vi "Prase XML.vi"() -> ()   [LabVIEW 2020]
uses:
  <vilib>/xml/Close Reference(Node).vi
  <vilib>/xml/Close Reference(NdList).vi
  <vilib>/xml/NI_XML.lvlib
  <resource>/objmgr/DOMUserDefRef.rc
panel:
  out "Test\nConfiguration":T1(array[cluster])
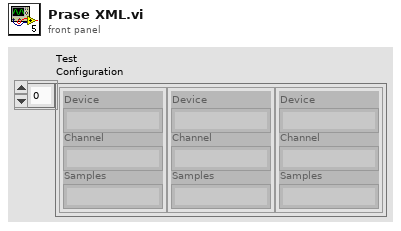
[diagram p1: front panel]
types:
  T1 = cluster{"Device":string, "Channel":string, "Samples":string}[]
  T2 = cluster{"Device":string, "Channel":string, "Samples":string}
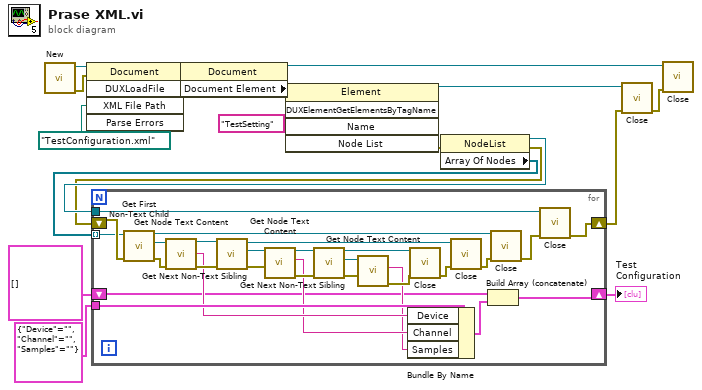
[diagram p0: block diagram]
diagram:
  n1 = call <vilib>:"New.vi"() -> ("error out"=w19:errorcluster, "DOM document out"=w20:refnum<k20>)  [unwired: 1 in, 7 out]
  n2 = invoke class="Document" method="DUXLoadFile"(reference=w20, error in=w19, "XML File Path"=path "TestConfiguration.xml") -> (reference out=w18:refnum<k20>, error out=w17:errorcluster)  [unwired: 2 in, 3 out]
  n3 = property class="Document"(reference=w18, error in=w17) -> (reference out=w6:refnum<k20>, error out=w15:errorcluster, "Document Element"=w7:refnum<k20>)
  n4 = invoke class="Element" method="DUXElementGetElementsByTagName"(reference=w7, error in=w15, "Name"="TestSetting" ("Node Name")) -> (reference out=w8:refnum<k20>, error out=w5:errorcluster, "Node List"=w4:refnum<k20>)  [unwired: 2 in, 2 out]
  n5 = property class="NodeList"(reference=w4, error in=w5) -> (reference out=w11:refnum<k20>, error out=w10:errorcluster, "Array Of Nodes"=w12:refnum<k20>[])
  n6 = for {
    tunnel: w12 -> [w21] mode=indexing
    tunnel: w11 -> [w32]
    shift-right: [w24] -> w1
    shift-left: T1 [] -> [w26]
    shift-right: [w31] -> w3
    shift-left: w10 -> [w23]
    tunnel: T2 {"Device"="", "Channel"="", "Samples"=""} -> [w30]
    n7 = call <vilib>:"Get First Non-Text Child.vi"("error in (no error)"=w23, "node in"=w21) -> ("error out"=w47:errorcluster, "child node"=w48:refnum<k20>, "node out"=w40:refnum<k20>)  [unwired: 7 out]
    n8 = call <vilib>:"Get Node Text Content.vi"("error in (no error)"=w47, "node in"=w48) -> ("error out"=w43:errorcluster, "node text"=w29:string, "node out"=w44:refnum<k20>)  [unwired: 7 out]
    n9 = call <vilib>:"Get Next Non-Text Sibling.vi"("error in (no error)"=w43, "node in"=w44) -> ("error out"=w46:errorcluster, "sibling node"=w45:refnum<k20>, "node out"=w42:refnum<k20>)  [unwired: 7 out]
    n10 = call <vilib>:"Get Node Text Content.vi"("error in (no error)"=w46, "node in"=w45) -> ("error out"=w36:errorcluster, "node text"=w28:string, "node out"=w38:refnum<k20>)  [unwired: 7 out]
    n11 = call <vilib>:"Get Next Non-Text Sibling.vi"("error in (no error)"=w36, "node in"=w38) -> ("error out"=w35:errorcluster, "sibling node"=w34:refnum<k20>, "node out"=w37:refnum<k20>)  [unwired: 7 out]
    n12 = call <vilib>:"Get Node Text Content.vi"("error in (no error)"=w35, "node in"=w34) -> ("error out"=w33:errorcluster, "node text"=w27:string)  [unwired: 8 out]
    n13 = Bundle By Name(cluster=w30, "Device"=w29, "Channel"=w28, "Samples"=w27) -> (w25:T2)
    n14 = call-poly <vilib>:"Close.vi"("error in (no error)"=w33, "node"=w37) -> ("error out"=w41:errorcluster)  [unwired: 7 out]
    n15 = call-poly <vilib>:"Close.vi"("error in (no error)"=w41, "node"=w42) -> ("error out"=w39:errorcluster)  [unwired: 7 out]
    n16 = Build Array (concatenate)(w26, w25) -> (w24:T1)
    n17 = call-poly <vilib>:"Close.vi"("error in (no error)"=w39, "node"=w40) -> ("error out"=w22:errorcluster)  [unwired: 7 out]
    n18 = call-poly <vilib>:"Close.vi"("error in (no error)"=w22, "node list"=w32) -> ("error out"=w31:errorcluster)  [unwired: 7 out]
  }
  "Test\nConfiguration" <- w1
  n19 = call-poly <vilib>:"Close.vi"("error in (no error)"=w3, "node"=w8) -> ("error out"=w9:errorcluster)  [unwired: 7 out]
  n20 = call-poly <vilib>:"Close.vi"("error in (no error)"=w9, "node"=w6) -> ()  [unwired: 8 out]
